vi "test.Runner.helper.vi"(11 "Parameters.in":T2) -> (0 "error out":errorcluster, 3 "Results.out":T1)   [LabVIEW 2020]
panel:
  out "Results (live)":cluster{"Test Vi":string, "Passed?":bool}[](array[cluster])
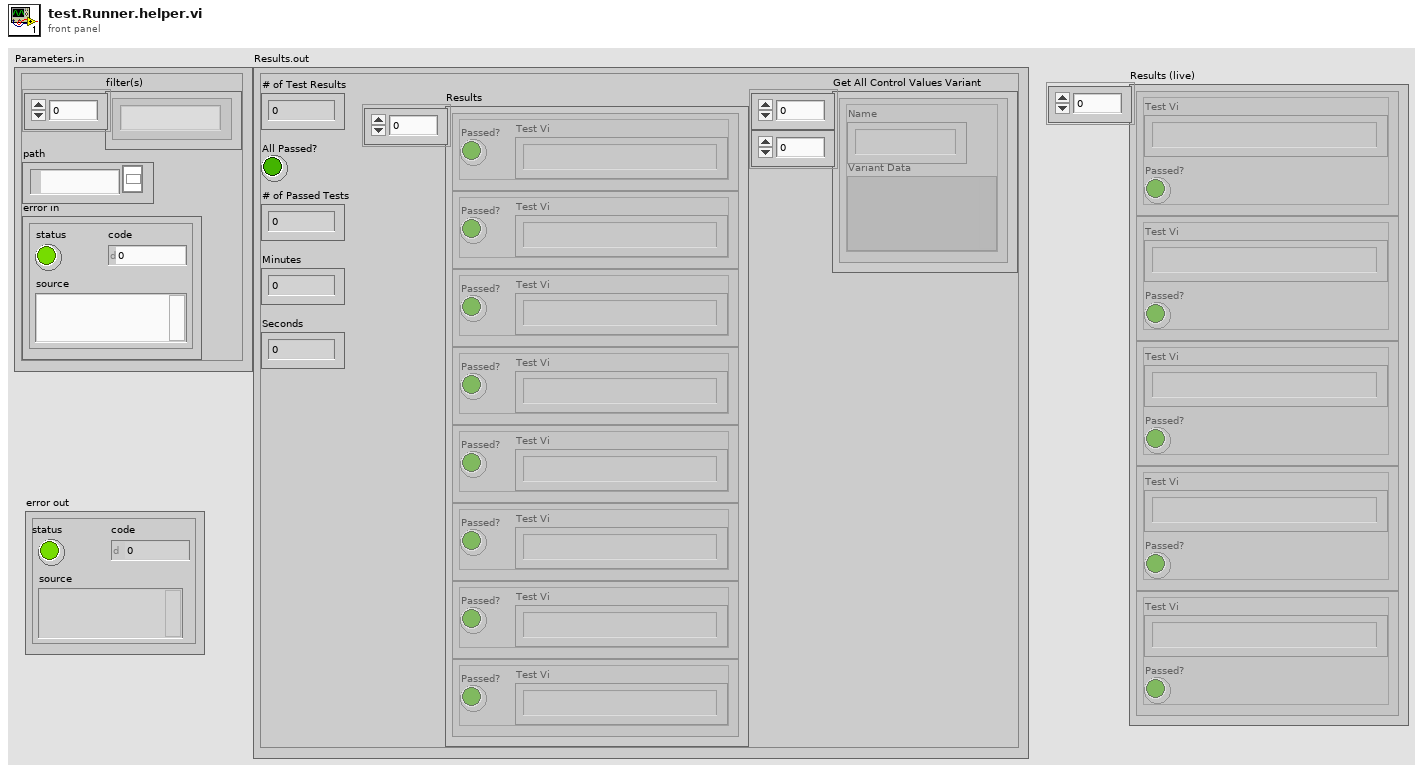
[diagram p1: front panel]
types:
  T1 = cluster{"Results":cluster{"Test Vi":string, "Passed?":bool}[], "# of Test Results":i32, "All Passed?":bool, "# of Passed Tests":i32, "Minutes":u32, "Seconds":u32, "Get All Control Values Variant":cluster{"Name":string, "Variant Data":variant}[][]}
  T2 = cluster{"filter(s)":string[], "path":path, "error in":errorcluster}
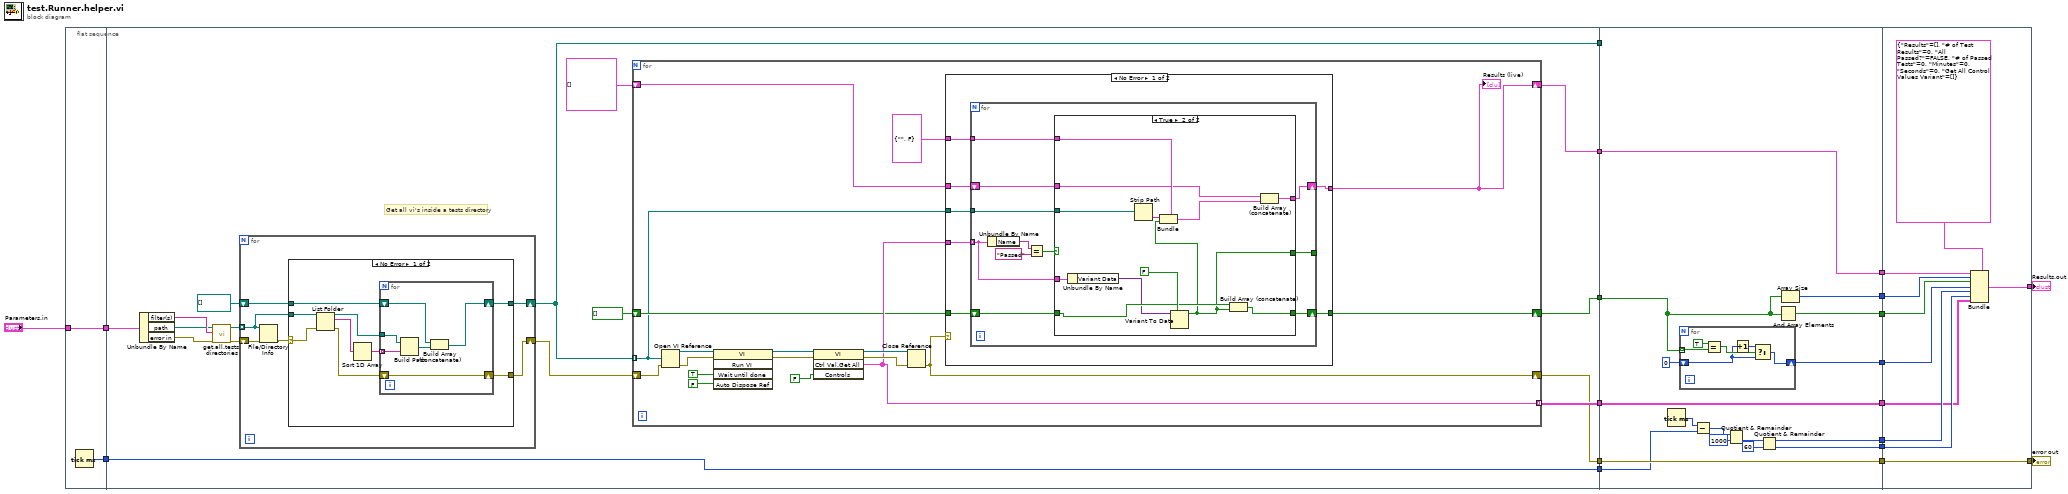
[diagram p0: block diagram]
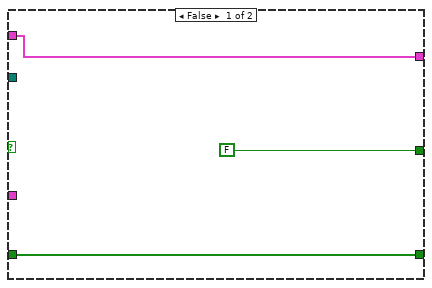
[diagram p3: hidden frame]
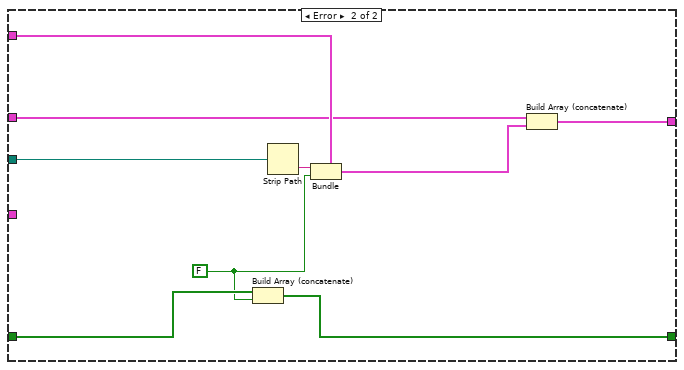
[diagram p4: hidden frame]
diagram:
  n1 = flat-sequence {
    tunnel: "Parameters.in" -> [w21]
    tunnel: [w21] -> w19
    tunnel: [w20] -> w18
    tunnel: [w37] -> w17
    tunnel: [w25] -> w16
    tunnel: [w36] -> w15
    tunnel: [w35] -> w14
    tunnel: w19 -> [w31]
    tunnel: w18 -> [w26]
    tunnel: [w26] -> w13
    tunnel: [w22] -> w1
    tunnel: w17 -> [_]
    tunnel: w16 -> [w136]
    tunnel: w15 -> [w123]
    tunnel: w14 -> [w131]
    tunnel: [w134] -> w12
    tunnel: [w133] -> w11
    tunnel: [w132] -> w10
    tunnel: [w121] -> w9
    tunnel: [w131] -> w8
    tunnel: [w125] -> w7
    tunnel: [w124] -> w6
    tunnel: [w123] -> w5
    tunnel: w13 -> [w122]
    tunnel: w1 -> [w121]
    tunnel: w12 -> [w149]
    tunnel: w11 -> [w150]
    tunnel: w10 -> [w151]
    tunnel: w9 -> [w152]
    tunnel: w8 -> [w143]
    tunnel: w7 -> [w147]
    tunnel: w6 -> [w148]
    tunnel: w5 -> [w146]
    tunnel: [w144] -> w2
    tunnel: [w143] -> w4
    frame #0 {
      n2 = Tick Count (ms)() -> (millisecond timer value=w20:u32)
    }
    frame #1 {
      # "Get all vi's inside a tests directory"
      n3 = Unbundle By Name(w31) -> ("filter(s)"=w30:string[], "path"=w29:path, "error in"=w28:errorcluster)
      n4 = call "get.all.tests.directories.vi"("error in"=w28, "filter(s)"=w30, "Path.in"=w29) -> ("error out"=w27:errorcluster, "Test Directories"=w33:path[])  [unwired: 7 in]
      n5 = for {
        tunnel: w33 -> [w42] mode=indexing
        shift-right: [w40] -> w37
        shift-left: path[] [] -> [w41]
        shift-right: [w38] -> w34
        shift-left: w27 -> [w39]
        n6 = File/Directory Info(path=w42, error in=w39) -> (error out=w43:errorcluster)  [unwired: 6 out]
        n7 = case shown="No Error" w43 {
          selector: w43 -> [w51 w60]
          tunnel: w42 -> [w52 _]
          tunnel: [w48 w60] -> w38
          tunnel: [w45 w59] -> w40
          tunnel: w41 -> [w44 w59]
          frame No Error {
            n8 = List Folder(path=w52, error in=w51) -> (path out=w50:path, filenames=w47:string[], error out=w49:errorcluster)  [unwired: 2 in, 1 out]
            n9 = Sort 1D Array(array=w47) -> (sorted array=w46:string[])
            n10 = for {
              tunnel: w50 -> [w58]
              shift-right: [w53] -> w48
              shift-left: w49 -> [w53]
              tunnel: w46 -> [w57] mode=indexing
              shift-right: [w55] -> w45
              shift-left: w44 -> [w54]
              n11 = Build Path(base path=w58, name or relative path=w57) -> (appended path=w56:path)
              n12 = Build Array (concatenate)(w54, w56) -> (w55:path[])
            }
          }
          frame Error {
          }
        }
      }
      n13 = for {
        tunnel: [w67] -> w36 mode=indexing
        tunnel: w37 -> [w63] mode=indexing
        shift-right: [w68] -> w35
        shift-left: w34 -> [w69]
        shift-right: [w66] -> w25
        shift-left: bool[] [] -> [w65]
        shift-right: [w62] -> w22
        shift-left: cluster{"Test Vi":string, "Passed?":bool}[] [] -> [w61]
        n14 = Open VI Reference(vi path=w63, error in (no error)=w69) -> (vi reference=w78:refnum<vi>, error out=w77:errorcluster)  [unwired: 4 in]
        n15 = invoke class="VI" method="Run VI"(reference=w78, error in=w77, "Wait until done"=TRUE ("Wait Until Done"), "Auto Dispose Ref"=FALSE ("Auto Dispose Reference")) -> (reference out=w76:refnum<vi>, error out=w71:errorcluster)  [unwired: 1 in, 3 out]
        n16 = invoke class="VI" method="Ctrl Val.Get All"(reference=w76, error in=w71, "Controls"=FALSE) -> (reference out=w72:refnum<vi>, error out=w70:errorcluster, "Get All Control Values Variant"=w67:cluster{"Name":string, "Variant Data":variant}[])  [unwired: 1 in, 1 out]
        n17 = Close Reference(reference=w72, error in (no error)=w70) -> (error out=w68:errorcluster)
        n18 = case shown="No Error" w68 {
          tunnel: w67 -> [w85 _]
          tunnel: [w84 w119] -> w66
          tunnel: w65 -> [w83 w120]
          tunnel: cluster{"Test Vi":string, "Passed?":bool} {"Test Vi"="", "Passed?"=FALSE} ("cluster") -> [w81 w117]
          tunnel: w63 -> [w82 w116]
          tunnel: [w79 w113] -> w62
          tunnel: w61 -> [w80 w112]
          frame No Error {
            n19 = for {
              tunnel: w85 -> [w93] mode=indexing
              shift-right: [w91] -> w84
              shift-left: w83 -> [w92]
              tunnel: [w90] -> _
              tunnel: w82 -> [w89]
              tunnel: w81 -> [w88]
              shift-right: [w86] -> w79
              shift-left: w80 -> [w87]
              n20 = Unbundle By Name(w93) -> ("Name"=w96:string)
              n21 = Equal?(x=w96, y="Passed") -> (x = y?=w94:bool)
              n22 = case shown="True" w94 {
                tunnel: w93 -> [_ w111]
                tunnel: [w99 w109] -> w91
                tunnel: w92 -> [w99 w108]
                tunnel: [FALSE w104] -> w90
                tunnel: w89 -> [_ w105]
                tunnel: w88 -> [_ w103]
                tunnel: [w97 w101] -> w86
                tunnel: w87 -> [w97 w100]
                frame False {
                }
                frame True {
                  n23 = Unbundle By Name(w111) -> ("Variant Data"=w107:variant)
                  n24 = Strip Path(path=w105) -> (name=w106:string)  [unwired: 1 out]
                  n25 = Variant To Data(type=FALSE, Variant=w107) -> (data=w104:bool)  [unwired: 1 in, 1 out]
                  n26 = Bundle(cluster=w103, "Test Vi"=w106, "Passed?"=w104) -> (w102:cluster{"Test Vi":string, "Passed?":bool})
                  n27 = Build Array (concatenate)(w108, w104) -> (w109:bool[])
                  n28 = Build Array (concatenate)(w100, w102) -> (w101:cluster{"Test Vi":string, "Passed?":bool}[])
                }
              }
            }
          }
          frame Error {
            w115 = FALSE
            n29 = Build Array (concatenate)(w120, w115) -> (w119:bool[])
            n30 = Strip Path(path=w116) -> (name=w118:string)  [unwired: 1 out]
            n31 = Bundle(cluster=w117, "Test Vi"=w118, "Passed?"=w115) -> (w114:cluster{"Test Vi":string, "Passed?":bool})
            n32 = Build Array (concatenate)(w112, w114) -> (w113:cluster{"Test Vi":string, "Passed?":bool}[])
          }
        }
        "Results (live)" <- w62
      }
    }
    frame #2 {
      n33 = Tick Count (ms)() -> (millisecond timer value=w128:u32)
      n34 = for {
        tunnel: w136 -> [w142] mode=indexing
        shift-right: [w139] -> w134
        shift-left: 0 -> [w138]
        n35 = Equal?(x=TRUE, y=w142) -> (x = y?=w140:bool)
        n36 = Increment(x=w138) -> (x+1=w137:i32)
        n37 = Select(t=w137, s=w140, f=w138) -> (s? t:f=w139:i32)
      }
      n38 = Subtract(x=w128, y=w122) -> (x-y=w129:u32)
      n39 = Quotient & Remainder(x=w129, y=u32 1000) -> (floor(x/y)=w130:u32)  [unwired: 1 out]
      n40 = Quotient & Remainder(x=w130, y=u32 60) -> (x-y*floor(x/y)=w124:u32, floor(x/y)=w125:u32)
      n41 = And Array Elements(Boolean array=w136) -> (logical AND=w133:bool)
      n42 = Array Size(array=w136) -> (size(s)=w132:i32)
    }
    frame #3 {
      n43 = Bundle(cluster=T1 {"Results"=[], "# of Test Results"=0, "All Passed?"=FALSE, "# of Passed Tests"=0, "Minutes"=0, "Seconds"=0, "Get All Control Values Variant"=[]}, "Results"=w152, "# of Test Results"=w151, "All Passed?"=w150, "# of Passed Tests"=w149, "Minutes"=w148, "Seconds"=w147, "Get All Control Values Variant"=w146) -> (w144:T1)
    }
  }
  "error out" <- w4
  "Results.out" <- w2
